vi "Teleop.vi"(10 "Match Info":T1={"Autonomous Elapsed Seconds"=0.0, "TeleOp Elapsed Seconds"=0.0, "Disabled Elapsed Seconds"=0.0, "Visited Autonomous"=FALSE, "Visited TeleOp"=FALSE, "Visited Disabled"=FALSE, "Autonomous Settings"={"Autonomous Style"=enum."Independent", "VI Refnum"=refnum}}, 11 "Call Context":T2) -> ()   [LabVIEW 2019]
doc: "This VI is called for each TeleOp packet received from the DS where the robot is not disabled. It is often used to read from the joysticks and update I/O or to update setpoints for timed control loops. It should complete and return within 20 milliseconds or it may miss DS packets."
uses:
  <vilib>/Rock Robotics/WPI/DriverStation/WPI_DriverStationDerivedRobotMode.ctl
  <vilib>/Rock Robotics/WPI/DriverStation/WPI_DriverStationMatch Info.ctl
  Robot Global Data.vi
  <vilib>/Rock Robotics/Network Tables/NT Write Number.vi
  <vilib>/Rock Robotics/WPI/Utilities/WPI_GetSetVariantRefNum.vi
panel:
  in  "Chassis X SPD":dbl=0.65
  in  "Chassis Y SPD":dbl=0.65
  # "Click here to set max"
  # "Click here to set min"
  # "Click here to set max"
  # "Click here to set min"
  # "Click here to set max"
  # "Click here to set min"
  # "Click here to set max"
  # "Click here to set min"
  # "Click here to set max"
  # "Click here to set min"
  # "Click here to set max"
  # "Click here to set min"
  # "Click here to set max"
  # "Click here to set min"
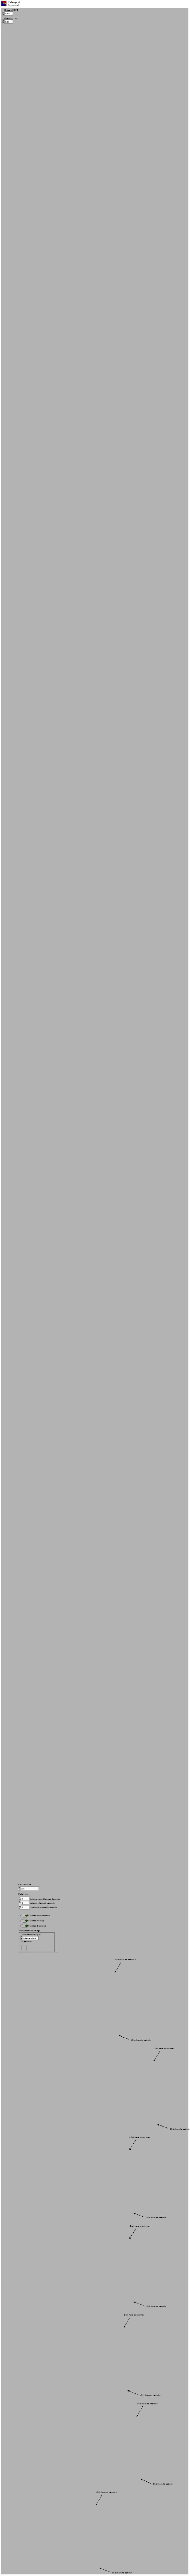
[diagram p1: front panel]
types:
  T1 = typedef "WPI_DriverStationMatch Info.ctl" = cluster{"Autonomous Elapsed Seconds":dbl, "TeleOp Elapsed Seconds":dbl, "Disabled Elapsed Seconds":dbl, "Visited Autonomous":bool, "Visited TeleOp":bool, "Visited Disabled":bool, "Autonomous Settings":cluster{"Autonomous Style":enum16{"Iterative", "Independent"}, "VI Refnum":refnum<vi>}}
  T2 = typedef "WPI_DriverStationDerivedRobotMode.ctl" = enum16{"Init", "Execute", "Stop"}
  T3 = typedef "WPI_MotorControlDeviceRef.ctl" = cluster{"DeviceStatus":errorcluster, "Type":T4, "PWM":cluster{"PWM Channel":T5, "DeadBand":T6}, "CAN":cluster{"Device Number":u8, "SetOutput VI Ref":variant, "GetOutput VI Ref":variant, "Enable VI Ref":variant, "Disable VI Ref":variant, "Data":variant}, "Invert":bool, "DIO PWM":cluster{"PWM \"Enable\" Channel":T5, "DIOChannel":T7, "PWM Rate":dbl}}
  T4 = typedef "WPI_MotorControlType.ctl" = enum16{"PWM", "CAN", "DIO PWM"}
  T5 = typedef "FPGA_DIOPWMChannel.ctl" = enum8{"PWM 0", "PWM 1", "PWM 2", "PWM 3", "PWM 4", "PWM 5", "PWM 6", "PWM 7", "PWM 8", "PWM 9", "PWM MXP 0", "PWM MXP 1", "PWM MXP 2", "PWM MXP 3", "PWM MXP 4", "PWM MXP 5", "PWM MXP 6", "PWM MXP 7", "PWM MXP 8", "PWM MXP 9", "Invalid"}
  T6 = typedef "WPI_PWMDeadband.ctl" = cluster{"Name":string, "maxPositivePwm":i32, "minPositivePwm":i32, "centerPwm":i32, "maxNegativePwm":i32, "minNegativePwm":i32, "angularRange":u16}
  T7 = typedef "FPGA_DIOChannel.ctl" = enum8{"DIO 0", "DIO 1", "DIO 2", "DIO 3", "DIO 4", "DIO 5", "DIO 6", "DIO 7", "DIO 8", "DIO 9", "DIO MXP 0", "DIO MXP 1", "DIO MXP 2", "DIO MXP 3", "DIO MXP 4", "DIO MXP 5", "DIO MXP 6", "DIO MXP 7", "DIO MXP 8", "DIO MXP 9", "DIO MXP 10", "DIO MXP 11", "DIO MXP 12", "DIO MXP 13", "DIO MXP 14", "DIO MXP 15", "SPI Port CS1", "SPI Port CS2", "SPI Port CS3", "SPI Port MISO", "SPI Port MOSI", "Invalid"}
  T8 = typedef "WPI_ServoDeviceRef.ctl" = cluster{"DeviceStatus":errorcluster, "PWM Channel":T5, "DeadBand":T6}
  T9 = typedef "WPI_JoystickDevRef.ctl" = cluster{"Device":T10}
  T10 = typedef "WPI_JoystickDeviceEnum.ctl" = enum16{"USB 0", "USB 1", "USB 2", "USB 3", "USB 4", "USB 5"}
  T11 = typedef "WPI_RobotDriveDevRef.ctl" = cluster{"DevStatus":errorcluster, "Motors[]":T3[], "Square Inputs":bool, "Max Output":dbl}
  T12 = cluster{"JoystickDevRef":T9, "RobotDriveDevRef":T11}
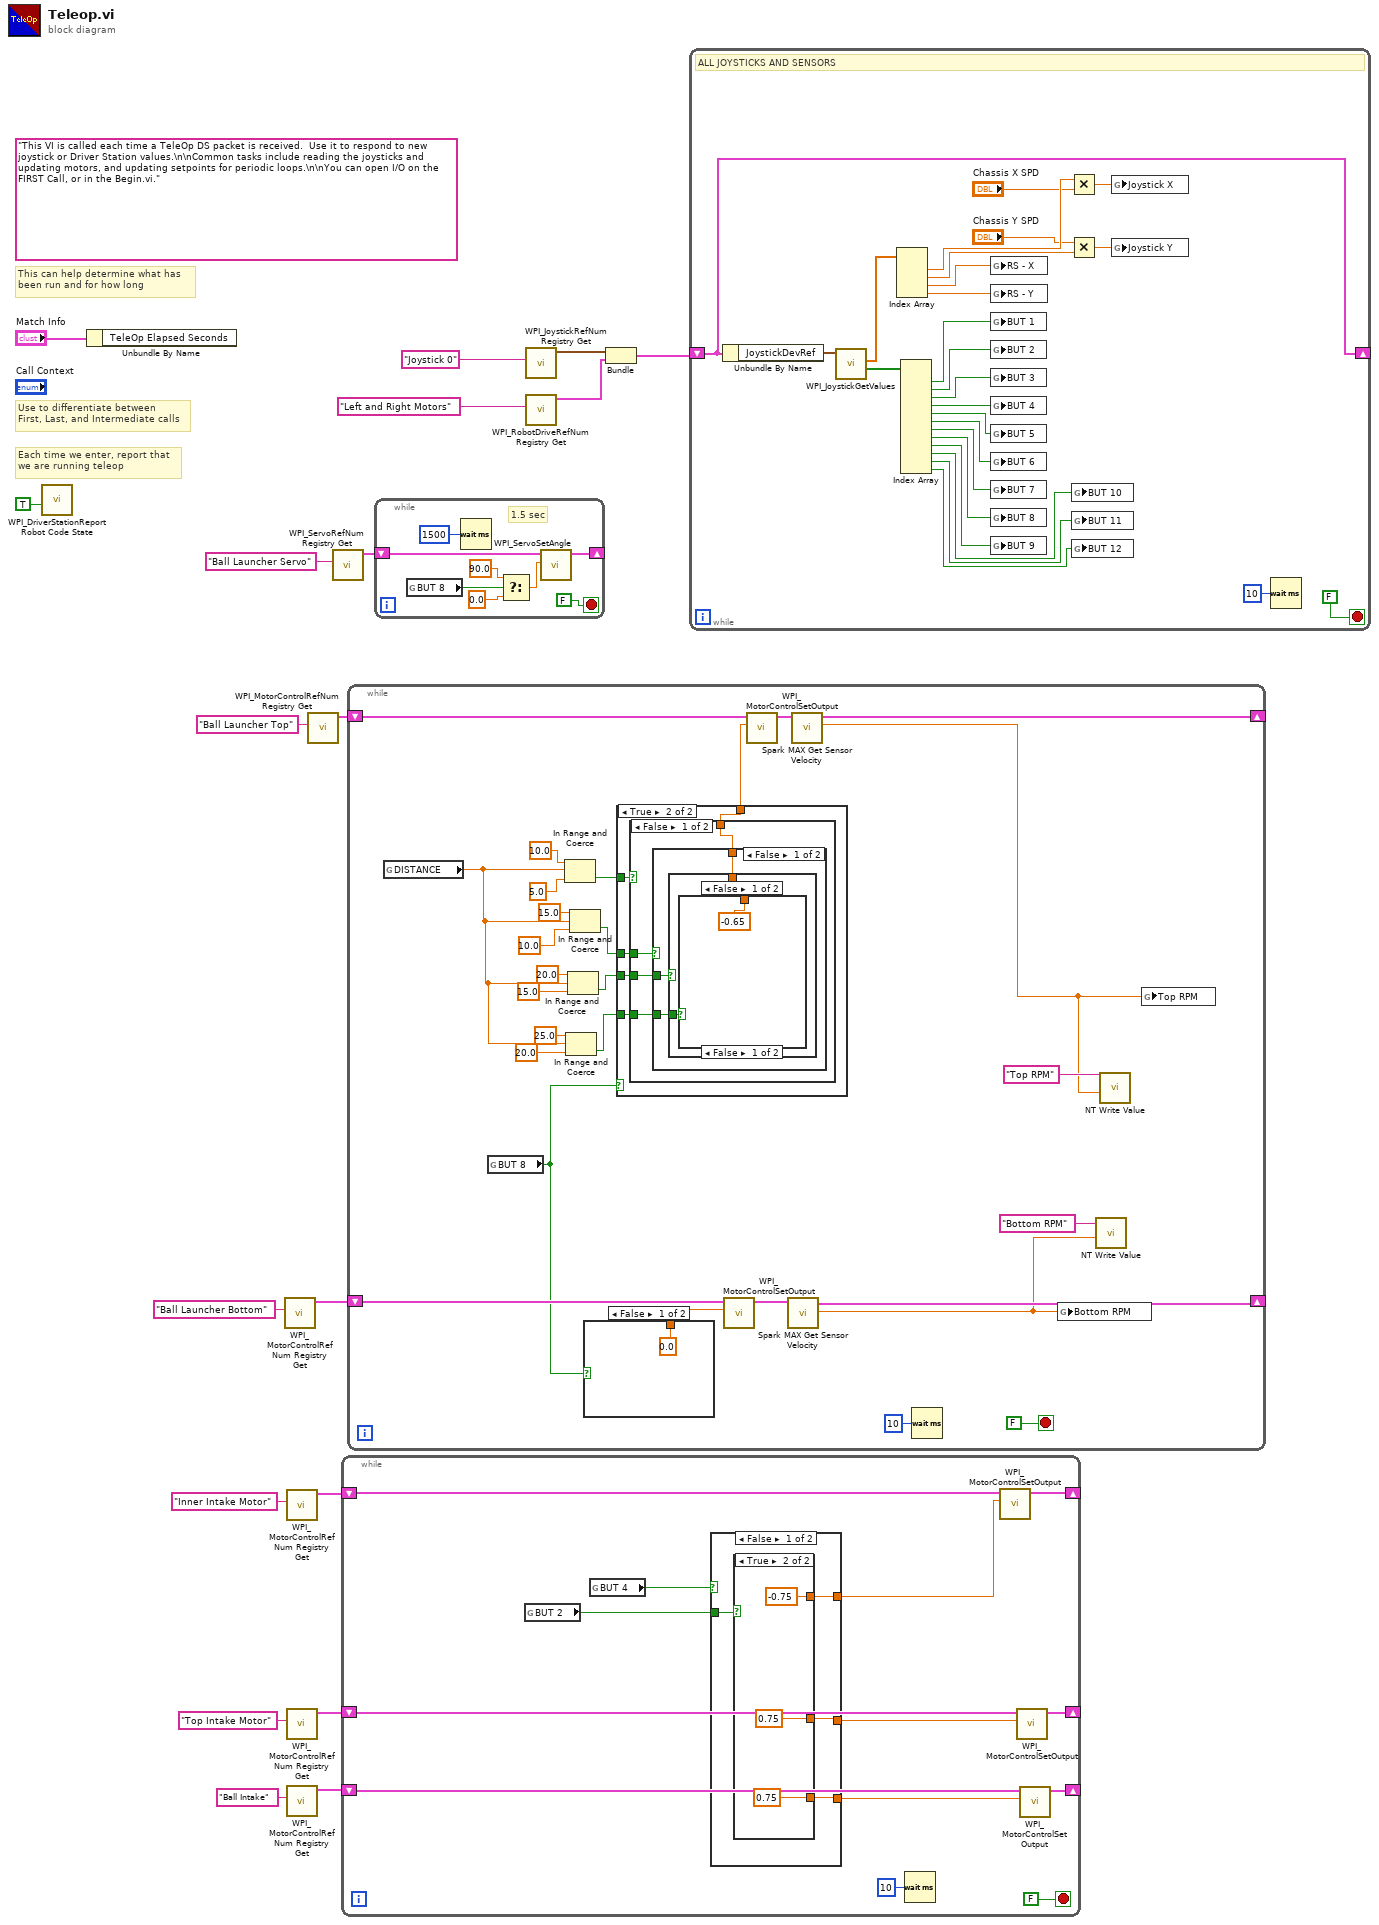
[diagram p0: block diagram]
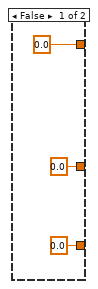
[diagram p2: hidden frame]
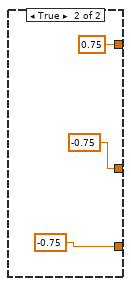
[diagram p3: hidden frame]
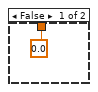
[diagram p4: hidden frame]
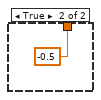
[diagram p5: hidden frame]
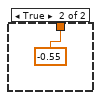
[diagram p6: hidden frame]
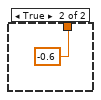
[diagram p7: hidden frame]
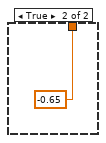
[diagram p8: hidden frame]
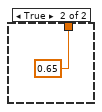
[diagram p9: hidden frame]
diagram:
  (unwired) "This VI is called each time a TeleOp DS packet is received.  Use it to respond to new joystick or Driver Station values.\n\nCommon tasks include reading the joysticks and updating motors, and updating setpoints for periodic loops.\n\nYou can open I/O on the FIRST Call, or in the Begin.vi."
  # "Each time we enter, report that\nwe are running teleop"
  # "Use to differentiate between\nFirst, Last, and Intermediate calls"
  # "This can help determine what has\nbeen run and for how long"
  n1 = call <vilib>:"WPI_DriverStationReport Robot Code State.vi"("TeleOp"=TRUE ("Autonomous")) -> ()  [unwired: 10 in, 1 out]
  n2 = Unbundle By Name("Match Info") -> ()  [unwired: 1 out]
  n3 = call <vilib>:"WPI_MotorControlRefNum Registry Get.vi"("refnum name"="Ball Launcher Bottom") -> ("MotorControlDevRef"=w12:T3)  [unwired: 9 in, 1 out]
  n4 = call <vilib>:"WPI_MotorControlRefNum Registry Get.vi"("refnum name"="Inner Intake Motor") -> ("MotorControlDevRef"=w10:T3)  [unwired: 9 in, 1 out]
  n5 = call <vilib>:"WPI_MotorControlRefNum Registry Get.vi"("refnum name"="Top Intake Motor") -> ("MotorControlDevRef"=w3:T3)  [unwired: 9 in, 1 out]
  n6 = call <vilib>:"WPI_MotorControlRefNum Registry Get.vi"("refnum name"="Ball Intake") -> ("MotorControlDevRef"=w1:T3)  [unwired: 9 in, 1 out]
  n7 = call <vilib>:"WPI_MotorControlRefNum Registry Get.vi"("refnum name"="Ball Launcher Top") -> ("MotorControlDevRef"=w15:T3)  [unwired: 9 in, 1 out]
  n8 = call <vilib>:"WPI_ServoRefNum Registry Get.vi"("refnum name"="Ball Launcher Servo") -> ("ServoDeviceRef"=w17:T8)  [unwired: 9 in, 1 out]
  n9 = while {
    shift-right: [w31] -> _
    shift-left: w10 -> [w30]
    shift-right: [w25] -> _
    shift-left: w3 -> [w26]
    shift-right: [w23] -> _
    shift-left: w1 -> [w22]
    stop <- FALSE stop-if-true
    n10 = global read "Robot Global Data.vi" "BUT 2"() -> (w29:bool)
    n11 = global read "Robot Global Data.vi" "BUT 4"() -> (w28:bool)
    n12 = case shown="False" w28 {
      tunnel: [w36 0.75 ("Output")] -> w24
      tunnel: w29 -> [w35 _]
      tunnel: [w34 -0.75 ("Output")] -> w21
      tunnel: [w33 -0.75 ("Output")] -> w20
      frame False {
        n13 = case shown="True" w35 {
          tunnel: [0.0 ("Output") -0.75 ("Output")] -> w36
          tunnel: [0.0 ("Output") 0.75 ("Output")] -> w34
          tunnel: [0.0 ("Output") 0.75 ("Output")] -> w33
          frame False {
          }
          frame True {
          }
        }
      }
      frame True {
      }
    }
    n14 = Wait (ms)(milliseconds to wait=u32 10) -> ()  [unwired: 1 out]
    n15 = call <vilib>:"WPI_MotorControlSetOutput.vi"("Output"=w24, "MotorControlDevRef"=w30) -> ("MotorControlDevRef"=w31:T3)  [unwired: 7 in, 2 out]
    n16 = call <vilib>:"WPI_MotorControlSetOutput.vi"("Output"=w21, "MotorControlDevRef"=w26) -> ("MotorControlDevRef"=w25:T3)  [unwired: 7 in, 2 out]
    n17 = call <vilib>:"WPI_MotorControlSetOutput.vi"("Output"=w20, "MotorControlDevRef"=w22) -> ("MotorControlDevRef"=w23:T3)  [unwired: 7 in, 2 out]
  }
  n18 = while {
    shift-right: [w60] -> _
    shift-left: w15 -> [w66]
    shift-right: [w69] -> _
    shift-left: w12 -> [w71]
    stop <- FALSE stop-if-true
    n19 = global read "Robot Global Data.vi" "DISTANCE"() -> (w47:dbl)
    n20 = global read "Robot Global Data.vi" "BUT 8"() -> (w46:bool)
    n21 = In Range and Coerce(upper limit=10.0, x=w47, lower limit=5.0) -> (In Range?=w59:bool)  [unwired: 1 out]
    n22 = In Range and Coerce(upper limit=25.0, x=w47, lower limit=20.0) -> (In Range?=w50:bool)  [unwired: 1 out]
    n23 = In Range and Coerce(upper limit=20.0, x=w47, lower limit=15.0) -> (In Range?=w53:bool)  [unwired: 1 out]
    n24 = In Range and Coerce(upper limit=15.0, x=w47, lower limit=10.0) -> (In Range?=w56:bool)  [unwired: 1 out]
    n25 = case shown="False" w46 {
      tunnel: [0.0 ("Output") 0.65 ("Output")] -> w68
      frame False {
      }
      frame True {
      }
    }
    n26 = case shown="True" w46 {
      tunnel: [0.0 ("Output") w79] -> w67
      tunnel: w59 -> [_ w78]
      tunnel: w56 -> [_ w77]
      tunnel: w53 -> [_ w76]
      tunnel: w50 -> [_ w75]
      frame False {
      }
      frame True {
        n27 = case shown="False" w78 {
          tunnel: [w80 -0.65 ("Output")] -> w79
          tunnel: w77 -> [w83 _]
          tunnel: w76 -> [w82 _]
          tunnel: w75 -> [w81 _]
          frame False {
            n28 = case shown="False" w83 {
              tunnel: w82 -> [w86 _]
              tunnel: w81 -> [w85 _]
              tunnel: [w84 -0.6 ("Output")] -> w80
              frame False {
                n29 = case shown="False" w86 {
                  tunnel: w85 -> [w88 _]
                  tunnel: [w87 -0.55 ("Output")] -> w84
                  frame False {
                    n30 = case shown="False" w88 {
                      tunnel: [-0.65 ("Output") -0.5 ("Output")] -> w87
                      frame False {
                      }
                      frame True {
                      }
                    }
                  }
                  frame True {
                  }
                }
              }
              frame True {
              }
            }
          }
          frame True {
          }
        }
      }
    }
    n31 = call <vilib>:"WPI_MotorControlSetOutput.vi"("Output"=w68, "MotorControlDevRef"=w71) -> ("MotorControlDevRef"=w70:T3)  [unwired: 7 in, 2 out]
    n32 = call <vilib>:"WPI_MotorControlSetOutput.vi"("Output"=w67, "MotorControlDevRef"=w66) -> ("MotorControlDevRef"=w65:T3)  [unwired: 7 in, 2 out]
    n33 = call <vilib>:"Spark MAX Get Sensor Velocity.vi"("MotorControlDevRef in"=w70) -> ("Sensor Velocity"=w61:dbl, "MotorControlDevRef out"=w69:T3)  [unwired: 7 in, 2 out]
    n34 = call <vilib>:"Spark MAX Get Sensor Velocity.vi"("MotorControlDevRef in"=w65) -> ("Sensor Velocity"=w63:dbl, "MotorControlDevRef out"=w60:T3)  [unwired: 7 in, 2 out]
    n35 = Wait (ms)(milliseconds to wait=u32 10) -> ()  [unwired: 1 out]
    n36 = global write "Robot Global Data.vi" "Bottom RPM"(w61) -> ()
    n37 = call-poly <vilib>:"NT Write Value.vi"("Numeric"=w61, "Name"="Bottom RPM") -> ()  [unwired: 9 in, 1 out]
    n38 = call-poly <vilib>:"NT Write Value.vi"("Numeric"=w63, "Name"="Top RPM") -> ()  [unwired: 9 in, 1 out]
    n39 = global write "Robot Global Data.vi" "Top RPM"(w63) -> ()
  }
  n40 = while {
    shift-right: [w99] -> _
    shift-left: w17 -> [w98]
    stop <- FALSE stop-if-true
    # "1.5 sec"
    n41 = global read "Robot Global Data.vi" "BUT 8"() -> (w96:bool)
    n42 = Wait (ms)(milliseconds to wait=u32 1500) -> ()  [unwired: 1 out]
    n43 = Select(t=90.0, s=w96, f=0.0) -> (s? t:f=w97:dbl)
    n44 = call <vilib>:"WPI_ServoSetAngle.vi"("Angle"=w97, "ServoDeviceRef"=w98) -> ("ServoDeviceRef"=w99:T8)  [unwired: 8 in, 1 out]
  }
  n45 = call <vilib>:"WPI_JoystickRefNum Registry Get.vi"("refnum name"="Joystick 0") -> ("JoystickDevRef"=w7:T9)  [unwired: 1 in, 9 out]
  n46 = call <vilib>:"WPI_RobotDriveRefNum Registry Get.vi"("refnum name"="Left and Right Motors") -> ("RobotDriveDevRef"=w6:T11)  [unwired: 1 in, 9 out]
  n47 = Bundle("JoystickDevRef"=w7, "RobotDriveDevRef"=w6) -> (w5:T12)  [unwired: 1 out]
  n48 = while {
    shift-right: [w114] -> _
    shift-left: w5 -> [w114]
    stop <- FALSE stop-if-true
    # "ALL JOYSTICKS AND SENSORS"
    n49 = Unbundle By Name(w114) -> ("JoystickDevRef"=w128:T9)
    n50 = call <vilib>:"WPI_JoystickGetValues.vi"("JoystickDevRef"=w128) -> ("Buttons"=w127:bool[], "Axes"=w113:dbl[])  [unwired: 6 in, 3 out]
    n51 = Index Array(array=w113) -> (element #1=w110:dbl, element #2=w109:dbl, element #3=w106:dbl, element #4=w105:dbl)  [unwired: 4 in]
    n52 = Index Array(array=w127) -> (element #1=w126:bool, element #2=w125:bool, element #3=w124:bool, element #4=w123:bool, element #5=w122:bool, element #6=w121:bool, element #7=w120:bool, element #8=w119:bool, element #9=w118:bool, element #10=w117:bool, element #11=w116:bool, element #12=w115:bool)  [unwired: 12 in]
    n53 = global write "Robot Global Data.vi" "RS - X"(w106) -> ()
    n54 = global write "Robot Global Data.vi" "RS - Y"(w105) -> ()
    n55 = global write "Robot Global Data.vi" "BUT 1"(w126) -> ()
    n56 = global write "Robot Global Data.vi" "BUT 2"(w125) -> ()
    n57 = global write "Robot Global Data.vi" "BUT 3"(w124) -> ()
    n58 = global write "Robot Global Data.vi" "BUT 4"(w123) -> ()
    n59 = global write "Robot Global Data.vi" "BUT 5"(w122) -> ()
    n60 = global write "Robot Global Data.vi" "BUT 6"(w121) -> ()
    n61 = global write "Robot Global Data.vi" "BUT 7"(w120) -> ()
    n62 = global write "Robot Global Data.vi" "BUT 8"(w119) -> ()
    n63 = global write "Robot Global Data.vi" "BUT 9"(w118) -> ()
    n64 = Multiply(x=w110, y="Chassis X SPD") -> (x*y=w112:dbl)
    n65 = Multiply(x="Chassis Y SPD", y=w109) -> (x*y=w111:dbl)
    n66 = global write "Robot Global Data.vi" "BUT 10"(w117) -> ()
    n67 = global write "Robot Global Data.vi" "BUT 11"(w116) -> ()
    n68 = global write "Robot Global Data.vi" "BUT 12"(w115) -> ()
    n69 = global write "Robot Global Data.vi" "Joystick X"(w112) -> ()
    n70 = global write "Robot Global Data.vi" "Joystick Y"(w111) -> ()
    n71 = Wait (ms)(milliseconds to wait=u32 10) -> ()  [unwired: 1 out]
  }
